vi "Activated TAsk.vi"(7 "Enum":enum16{"Read", "Write"}(ring), 8 "error in (no error)":errorcluster, 11 "Activate Task":T1={"Analog input"=TRUE, "Analog Output"=TRUE, "Digital input"=TRUE, "Digital output"=TRUE, "Thermocouple"=FALSE, "Strain Gauge"=TRUE, "Accelerometer"=TRUE}) -> (0 "error out":errorcluster, 1 "Start Time":timestamp, 2 "Activate Task 2":T1)   [LabVIEW 2022 SP3]
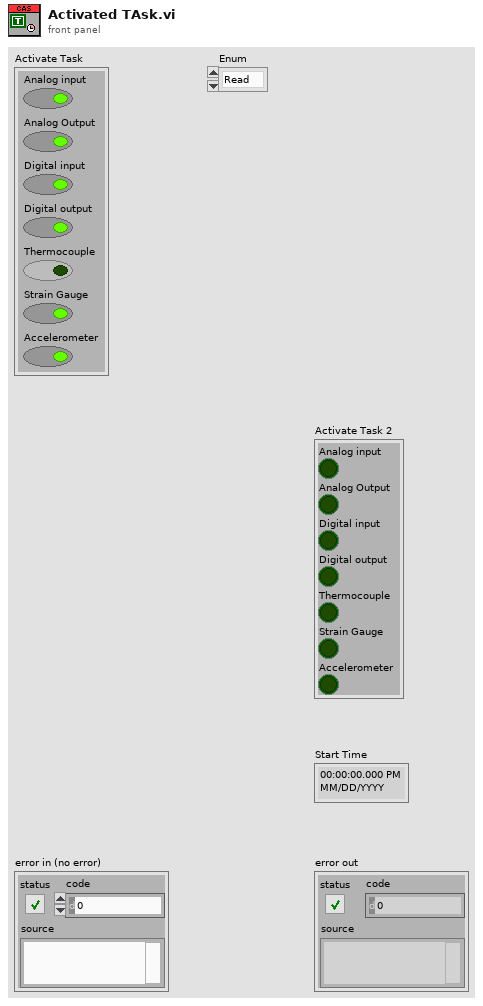
[diagram p1: front panel]
types:
  T1 = cluster{"Analog input":bool, "Analog Output":bool, "Digital input":bool, "Digital output":bool, "Thermocouple":bool, "Strain Gauge":bool, "Accelerometer":bool}
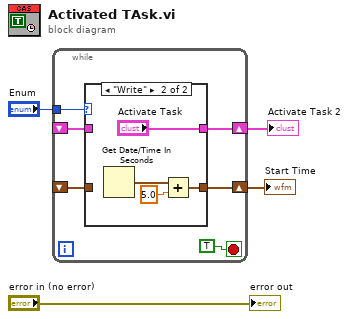
[diagram p0: block diagram]
diagram:
  n1 = while {
    tunnel: "Enum" -> [w10]
    shift-right: [w8] -> w3
    shift-left: _ -> [w7]
    shift-right: [w6] -> w1
    shift-left: _ -> [w5]
    stop <- TRUE stop-if-true
    n2 = case shown="\"Write\"" w10 {
      tunnel: [w12 w14] -> w8
      tunnel: w7 -> [w12 _]
      tunnel: [w11 "Activate Task"] -> w6
      tunnel: w5 -> [w11 _]
      frame "Read", Default {
      }
      frame "Write" {
        n3 = Get Date/Time In Seconds() -> (seconds since 1Jan1904=w16:timestamp)
        n4 = Add(x=w16, y=5.0) -> (x+y=w14:timestamp)
      }
    }
  }
  "Start Time" <- w3
  "Activate Task 2" <- w1
  "error out" <- "error in (no error)"
